vi "main.vi"() -> ()   [LabVIEW 2018]
uses:
  Program Files (x86)/National Instruments/LabVIEW 2018/examples/Instrument IO/Serial/support/Serial - Settings.ctl
  <vilib>/Instr/_visa.llb/VISA Configure Serial Port (Instr).vi
panel:
  in  "数据保存路径":path
  in  "RS485通讯":refnum<visa-resource-name>
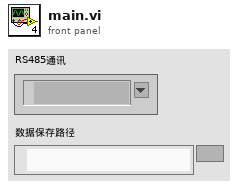
[diagram p1: front panel]
types:
  T1 = typedef "Serial - Settings.ctl" = cluster{"波特率":u32, "数据位":u16, "校验":enum16{"None", "Odd", "Even", "Mark", "Space"}, "停止位":u16, "流控制":u16}
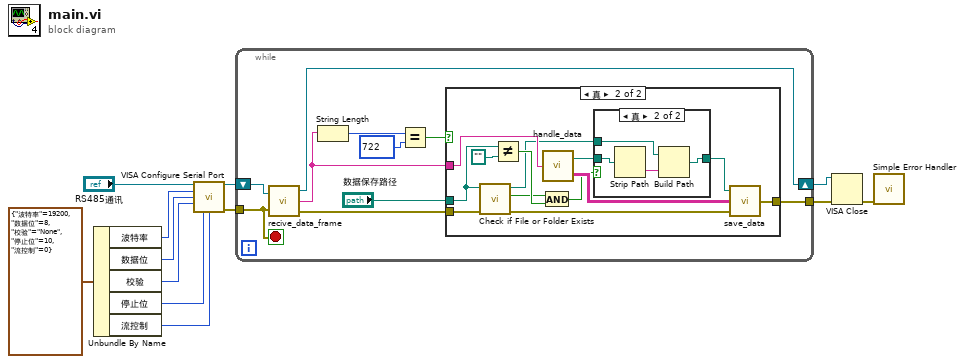
[diagram p0: block diagram]
diagram:
  n1 = Unbundle By Name(T1 {"波特率"=19200, "数据位"=8, "校验"=enum."None", "停止位"=10, "流控制"=0} ("输入簇")) -> ("波特率"=w11:u32, "数据位"=w10:u16, "校验"=w9:enum16{"None", "Odd", "Even", "Mark", "Space"}, "停止位"=w8:u16, "流控制"=w7:u16)
  n2 = call-poly "VISA Configure Serial Port"("VISA resource name"="RS485通讯", "baud rate (9600)"=w11, "data bits (8)"=w10, "parity (0:none)"=w9, "stop bits (10: 1 bit)"=w8, "flow control (0:none)"=w7) -> ("VISA resource name out"=w5:refnum<visa-resource-name>, "error out"=w4:errorcluster)  [unwired: 4 in, 4 out]
  n3 = while {
    tunnel: w4 -> [w13]
    tunnel: [w18] -> w2
    shift-right: [w16] -> w3
    shift-left: w5 -> [w22]
    stop <- w13 stop-if-true
    n4 = call "recive_data_frame.vi"("VISA resource name out"=w22, "错误输入（无错误）"=w13) -> ("VISA resource name out 2"=w16:refnum<visa-resource-name>, "字符串"=w15:string, "error out"=w17:errorcluster)
    n5 = String Length(string=w15) -> (length=w21:i32)
    n6 = Equal?(x=w21, y=722) -> (x = y?=w19:bool)
    n7 = case shown="真" w19 {
      tunnel: [w23 w34] -> w18
      tunnel: w17 -> [w23 w31]
      tunnel: w15 -> [_ w36]
      tunnel: "数据保存路径" -> [_ w28]
      frame False {
      }
      frame True {
        n8 = call <vilib>:"Check if File or Folder Exists.vi"("error in (no error)"=w31, "path"=w28) -> ("error out"=w30:errorcluster, "file or folder exists?"=w26:bool, "dup path"=w24:path)  [unwired: 7 in]
        n9 = Not Equal?(x=w28, y=path "") -> (x != y?=w27:bool)
        n10 = And(x=w26, y=w27) -> (x .and. y?=w25:bool)
        n11 = call "handle_data.vi"("串口数据"=w36) -> ("数据文件路径"=w33:path, "解析数据"=w35:string[][])
        n12 = case shown="真" w25 {
          tunnel: w33 -> [w37 w41]
          tunnel: w24 -> [_ w40]
          tunnel: [w37 w38] -> w32
          frame False {
          }
          frame True {
            n13 = Strip Path(path=w41) -> (name=w39:string)  [unwired: 1 out]
            n14 = Build Path(base path=w40, name or relative path=w39) -> (appended path=w38:path)
          }
        }
        n15 = call "save_data.vi"("error in (no error)"=w30, "Data"=w35, "数据文件路径"=w32) -> ("error out"=w34:errorcluster)
      }
    }
  }
  n16 = VISA Close(VISA resource name=w3, error in (no error)=w2) -> (error out=w1:errorcluster)
  n17 = call <vilib>:"Simple Error Handler.vi"("error in (no error)"=w1) -> ()  [unwired: 1 in, 8 out]
